vi "Accelerator Not Complex Process.vi"(9 "Sessions Parameters":T2={"intra_op_num_threads"=0, "inter_op_num_threads"=0, "execution_mode"=enum."ORT_SEQUENTIAL", "deterministic_compute"=FALSE, "graph_optimization_level"=1, "optimized_model_file_path"=path "", "profiling output dir"=path ""} {"graph_optimization_level" items=["ORT_DISABLE_ALL"=0, "ORT_ENABLE_ALL"=1, "ORT_ENABLE_BASIC"=2, "ORT_ENABLE_EXTENDED"=99]}, 10 "Execution Device":T1=enum."CUDA", 11 "X size":i32=16384) -> (3 "Accelerator Time":dbl=1.5238084999999728)   [LabVIEW 2020]
uses:
  Source/_Controls/acc_execution_provider_enum.ctl
  Source/ONNX/_Controls/acc_CUDA_ep_params_simplified.ctl
  Source/ONNX/_Controls/acc_tensorRT_ep_params_simplified.ctl
  Source/ONNX/Inference/acc_Inference.lvclass/acc_Inference.ctl
  Source/ONNX/Inference/_Methods/Simplified/acc_embedded_run_preallocated_multi_input_and_outputs_gpu_by_idx.vi
  Source/ONNX/Inference/_Methods/Simplified/acc_embedded_copy_ptr_data_to_labview_data.vi
  Source/ONNX/Inference/_Methods/Simplified/acc_embedded_run_mono_output_scalar_float.vi
  Source/SubVIs/sort_array/acc_sort_1d_index_ptr_data_cluster_array.vi
  Source/ONNX/Inference/_Methods/acc_embedded_run_preallocated_inputs_outputs_cuda_store_local.vi
  Source/SubVIs/sort_array/acc_sort_1d_index_out_ptr_data_cluster_array.vi
  Source/SubVIs/CUDAFunctions/acc_cuda_memcpy_device_to_host_bytes.vi
  Source/SubVIs/CUDAFunctions/acc_cuda_check_error.vi
  Source/SubVIs/CUDAFunctions/acc_cuda_error.vi
  Source/ONNX/Inference/acc_Inference.lvclass
  C:/Users/COCO/TDF Dropbox/1_Graiphic/3 - Services et Etudes/2 - Dev/code/Toolkits/Accelerator/Source/ONNX/acc_ONNX.lvclass
  Source/SubVIs/add_to_cluster_onnx_input/acc_onnx_add_1d_float_array_into_ptr_input_cluster_array_by_idx.vi
  Source/Model/_Methods/acc_create_onnx_model_then_init_cuda_inference_session.vi
  Source/Model/_Methods/acc_create_onnx_model_then_init_inference_session.vi
  Source/Model/_Methods/acc_create_onnx_model_then_init_tensorRT_inference_session.vi
  Source/SubVIs/add_to_cluster_onnx_input/acc_onnx_add_scalar_float_array_into_ptr_input_cluster_array_by_idx.vi
  Source/ONNX/Inference/_Methods/acc_embedded_check_execution_inputs_index.vi
  Source/ONNX/Inference/_Methods/acc_embedded_check_execution_outputs_index.vi
  Source/ONNX/_Accessors/acc_Read dll_path.vi
  Source/ONNX/SubVIs/acc_ONNX_CheckError.vi
  Source/SubVIs/CUDAFunctions/cuda_path_without_check_version.vi
  Source/SubVIs/Acc_ErrorStop.vi
  Source/SubVIs/checks/acc_check_output_onnx.vi
  Source/Model/acc_Model.lvclass
  <vilib>/Analysis/NI_AALBase.lvlib
panel:
  in  "nb_loop":i32=6
  out "max value":sgl=1.3257894e+20
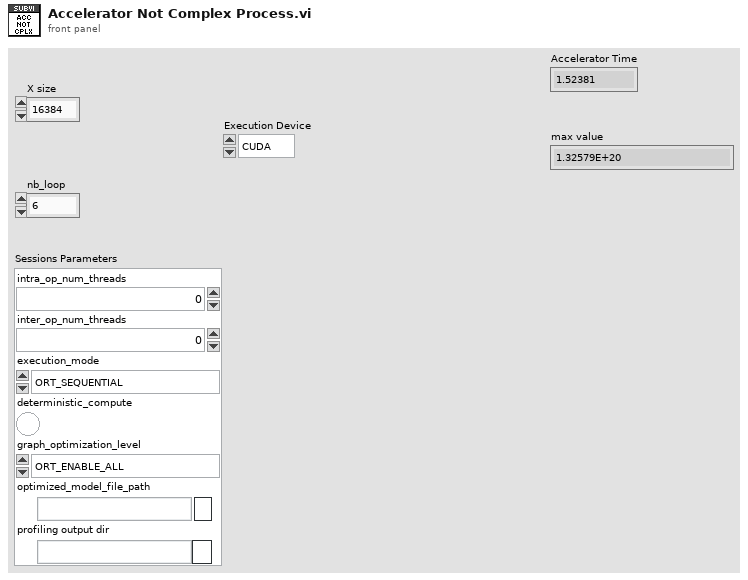
[diagram p1: front panel]
types:
  T1 = typedef "acc_execution_provider_enum.ctl" = enum16{"CPU", "CUDA", "TensorRT"}
  T2 = cluster{"intra_op_num_threads":i32, "inter_op_num_threads":i32, "execution_mode":enum16{"ORT_SEQUENTIAL", "ORT_PARALLEL"}, "deterministic_compute":bool, "graph_optimization_level":u16, "optimized_model_file_path":path, "profiling output dir":path}
  T3 = typedef "acc_onnx_multi_ptr_input_index_cluster.ctl" = cluster{"input_order":u32, "Inputs Info":cluster{"inputs_ptr":u64, "inputs_shapes":i64[], "inputs_ranks":i64, "inputs_types":T4}}
  T4 = typedef "acc_onnx_dtype_enum.ctl" = enum16{"UNDEFINED", "FLOAT", "UINT8", "INT8", "UINT16", "INT16", "INT32", "INT64", "STRING", "BOOL", "FLOAT16", "DOUBLE", "UINT32", "UINT64", "COMPLEX64", "COMPLEX128", "BFLOAT16", "FLOAT8E4M3FN", "FLOAT8E4M3FNUZ", "FLOAT8E5M2", "FLOAT8E5M2FNUZ", "UINT4", "INT4"}
  T5 = typedef "acc_CUDA_ep_params_simplified.ctl" = cluster{"Device & Stream":cluster{"Device Index":i32, "Use Custom Compute Stream?":bool, "Custom Compute Stream (Pointer)":u64, "Copy Using Default Stream?":bool}, "Memory Management":cluster{"GPU Memory Limit (Bytes)":u64, "Arena Extension Strategy":enum16{"kNextPowerOfTwo", "kSameAsRequested"}, "Default Memory Arena Config":u64}, "CuDNN & Kernel Optimization":cluster{"cuDNN Convolution Algorithm Search":enum16{"OrtCudnnConvAlgoSearchExhaustive", "OrtCudnnConvAlgoSearchHeuristic", "OrtCudnnConvAlgoSearchDefault"}, "Use Max Workspace for cuDNN?":bool, "Pad Conv1D Inputs to NC1D?":bool, "Fuse Convolution + Bias?":bool, "Scaled Dot-Product Attention Kernel Option":bool, "Enable Strict SkipLayerNorm Mode?":bool}, "Execution & Precision Controls":cluster{"Enable CUDA Graph Execution?":bool, "Use EP-Level Unified Stream?":bool, "Prefer NHWC Tensor Layout?":bool, "Use TensorFloat-32 (TF32)?":bool}, "Tunable Operator System":cluster{"Enable Tunable Operators?":bool, "Enable Tuning Mode for Tunable Operators?":bool, "Max Tuning Duration (ms)":i32}}
  T6 = typedef "acc_tensorRT_ep_params_simplified.ctl" = cluster{"Device And Stream":cluster{"Device Index":i32, "Use Custom Compute Stream?":bool, "Custom Compute Stream (Pointer)":u64}, "Parser & Subgraph Options":cluster{"Max Partition Attemps":i32, "Minimum Subgraph Size":i32}, "Memory & Workspace Management":cluster{"Max Workspace Memory (Bytes)":u64, "Share Memory Between Subgraphs":bool, "Auxiliary Stream Count":i32}, "Precision & Numeric Modes":cluster{"Enable FP16":bool, "Enable BF16":bool, "Enable INT8":bool, "INT8 Calibration Table Name":path, "Use Native INT8 Calibration?":bool}, "Engine Build, Cache & Paths":cluster{"Enable Engine Caching?":bool, "Engine Cache Directory":path, "Enable Engine Decryption?":bool, "Decryption Library Path":path, "Build Engines Sequentially?":bool, "Enable Timing Cache?":bool, "Timing Cache Directory":path, "Force Timing Cache Use?":bool, "Enable Detailed Logs?":bool, "Use Build Heuristics?":bool, "Enable Weight Sparsity?":bool, "Engine Optimization Level (0–5)":i32}, "Paths & Plugins":cluster{"Extra Plugin Libraries":path[], "Tactic Source Rules":string, "Enabled Preview Features":enum16{"None", "ALIASED_PLUGIN_IO_10_03"}}, "Profile Shapes":cluster{"Minimum Input Shapes":string, "Maximum Input Shapes":string, "Optimal Input Shapes":string}, "Advanced & DLA / CUDA Graph":cluster{"Enable DLA Acceleration?":bool, "DLA Core Index":i32, "Dump TensorRT Subgraphs?":bool, "Force LayerNorm in FP32?":bool, "Enable CUDA Graph Execution?":bool}}
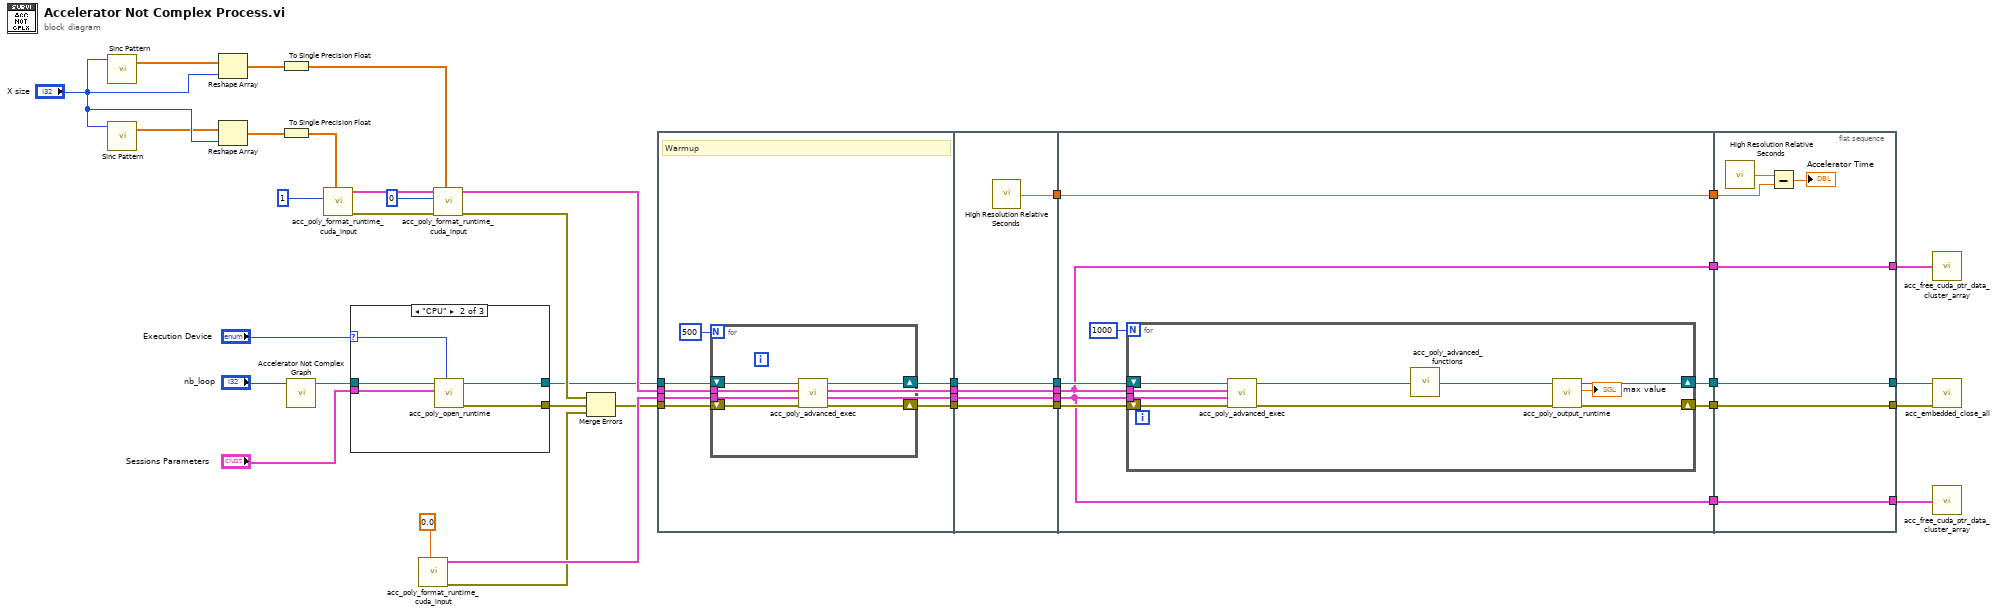
[diagram p0: block diagram]
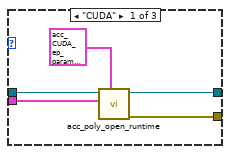
[diagram p2: hidden frame]
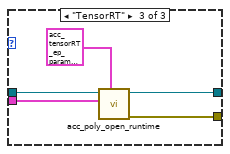
[diagram p3: hidden frame]
diagram:
  n1 = call <vilib>:"Sinc Pattern.vi"("samples"="X size") -> ("Sinc Pattern"=w8:dbl[])  [unwired: 3 in, 1 out]
  n2 = call <vilib>:"Sinc Pattern.vi"("samples"="X size") -> ("Sinc Pattern"=w9:dbl[])  [unwired: 3 in, 1 out]
  n3 = Reshape Array(w8, "X size") -> (w7:dbl[])
  n4 = Reshape Array(w9, "X size") -> (w6:dbl[])
  n5 = To Single Precision Float(number=w7) -> (single precision float=w10:sgl[])
  n6 = To Single Precision Float(number=w6) -> (single precision float=w11:sgl[])
  n7 = call "Accelerator Not Complex Graph.vi"("nb_loop"="nb_loop") -> ("Model out"=w3:refnum<class "acc_Model.lvclass">)  [unwired: 10 in]
  n8 = call-poly "acc_poly_format_runtime_cuda_input.vi"("1D Input Data"=w11, "input order"=1) -> ("error out"=w31:errorcluster, "Data in"=w36:T3[])  [unwired: 8 in]
  n9 = case shown="\"CPU\"" "Execution Device" {
    selector: "Execution Device" -> [_ w47 _]
    tunnel: [w46 w51 w56] -> w5
    tunnel: [w45 w50 w55] -> w1
    tunnel: "Sessions Parameters" -> [w44 w49 w54]
    tunnel: w3 -> [w43 w48 w53]
    frame "CUDA" {
      n10 = call-poly "acc_poly_open_runtime.vi"("CUDA Parameters"=T5 {"Device & Stream"={"Device Index"=0, "Use Custom Compute Stream?"=FALSE, "Custom Compute Stream (Pointer)"=0, "Copy Using Default Stream?"=TRUE}, "Memory Management"={"GPU Memory Limit (Bytes)"=18446744073709551615, "Arena Extension Strategy"=enum."kSameAsRequested", "Default Memory Arena Config"=0}, "CuDNN & Kernel Optimization"={"cuDNN Convolution Algorithm Search"=enum."OrtCudnnConvAlgoSearchHeuristic", "Use Max Workspace for cuDNN?"=FALSE, "Pad Conv1D Inputs to NC1D?"=FALSE, "Fuse Convolution + Bias?"=FALSE, "Scaled Dot-Product Attention Kernel Option"=FALSE, "Enable Strict SkipLayerNorm Mode?"=FALSE}, "Execution & Precision Controls"={"Enable CUDA Graph Execution?"=TRUE, "Use EP-Level Unified Stream?"=FALSE, "Prefer NHWC Tensor Layout?"=FALSE, "Use TensorFloat-32 (TF32)?"=TRUE}, "Tunable Operator System"={"Enable Tunable Operators?"=FALSE, "Enable Tuning Mode for Tunable Operators?"=FALSE, "Max Tuning Duration (ms)"=0}}, "Sessions Parameters"=w44, "Model in"=w43) -> ("error out"=w45:errorcluster, "Inference out"=w46:refnum<class "acc_Inference.lvclass">)  [unwired: 7 in]
    }
    frame "CPU" {
      n11 = call-poly "acc_poly_open_runtime.vi"("Execution Device"=w47, "Sessions Parameters"=w49, "Model in"=w48) -> ("error out"=w50:errorcluster, "Inference out"=w51:refnum<class "acc_Inference.lvclass">)  [unwired: 7 in]
    }
    frame "TensorRT" {
      n12 = call-poly "acc_poly_open_runtime.vi"("TRT Parameters"=T6 {"Device And Stream"={"Device Index"=0, "Use Custom Compute Stream?"=FALSE, "Custom Compute Stream (Pointer)"=0}, "Parser & Subgraph Options"={"Max Partition Attemps"=1000, "Minimum Subgraph Size"=1}, "Memory & Workspace Management"={"Max Workspace Memory (Bytes)"=0, "Share Memory Between Subgraphs"=FALSE, "Auxiliary Stream Count"=-1}, "Precision & Numeric Modes"={"Enable FP16"=FALSE, "Enable BF16"=FALSE, "Enable INT8"=FALSE, "INT8 Calibration Table Name"=path "", "Use Native INT8 Calibration?"=FALSE}, "Engine Build, Cache & Paths"={"Enable Engine Caching?"=FALSE, "Engine Cache Directory"=path "", "Enable Engine Decryption?"=FALSE, "Decryption Library Path"=path "", "Build Engines Sequentially?"=FALSE, "Enable Timing Cache?"=FALSE, "Timing Cache Directory"=path "", "Force Timing Cache Use?"=FALSE, "Enable Detailed Logs?"=FALSE, "Use Build Heuristics?"=FALSE, "Enable Weight Sparsity?"=FALSE, "Engine Optimization Level (0–5)"=3}, "Paths & Plugins"={"Extra Plugin Libraries"=[], "Tactic Source Rules"="", "Enabled Preview Features"=enum."None"}, "Profile Shapes"={"Minimum Input Shapes"="", "Maximum Input Shapes"="", "Optimal Input Shapes"=""}, "Advanced & DLA / CUDA Graph"={"Enable DLA Acceleration?"=FALSE, "DLA Core Index"=0, "Dump TensorRT Subgraphs?"=FALSE, "Force LayerNorm in FP32?"=FALSE, "Enable CUDA Graph Execution?"=FALSE}}, "Sessions Parameters"=w54, "Model in"=w53) -> ("error out"=w55:errorcluster, "Inference out"=w56:refnum<class "acc_Inference.lvclass">)  [unwired: 7 in]
    }
  }
  n13 = call-poly "acc_poly_format_runtime_cuda_input.vi"("Input Data"=sgl 0.0) -> ("error out"=w15:errorcluster, "Data in"=w34:T3[])  [unwired: 9 in]
  n14 = call-poly "acc_poly_format_runtime_cuda_input.vi"("1D Input Data"=w10, "error in"=w31, "input order"=0, "Data in"=w36) -> ("error out"=w16:errorcluster, "Data in"=w35:T3[])  [unwired: 6 in]
  n15 = Merge Errors(w16, w1, w15) -> (w29:errorcluster)
  n16 = flat-sequence {
    tunnel: w29 -> [w62]
    tunnel: w35 -> [w61]
    tunnel: w34 -> [w60]
    tunnel: [w63] -> w22
    tunnel: [w61] -> w21
    tunnel: [w60] -> w20
    tunnel: [w59] -> w19
    tunnel: w5 -> [w57]
    tunnel: [w74] -> w41
    tunnel: [w73] -> w39
    tunnel: [w72] -> w33
    tunnel: [w71] -> w32
    tunnel: [w70] -> w30
    tunnel: w22 -> [w73]
    tunnel: w21 -> [w71]
    tunnel: w20 -> [w72]
    tunnel: w19 -> [w70]
    tunnel: w41 -> [w82]
    tunnel: [w82] -> w40
    tunnel: w39 -> [w80]
    tunnel: w33 -> [w75]
    tunnel: w32 -> [w76]
    tunnel: w30 -> [w79]
    tunnel: [w78] -> w27
    tunnel: [w77] -> w26
    tunnel: [w76] -> w24
    tunnel: [w75] -> w23
    tunnel: w40 -> [w98]
    tunnel: [w96] -> w28
    tunnel: w27 -> [w96]
    tunnel: w26 -> [w95]
    tunnel: [w95] -> w25
    tunnel: [w94] -> w14
    tunnel: w24 -> [w94]
    tunnel: [w93] -> w13
    tunnel: w23 -> [w93]
    frame #0 {
      # "Warmup"
      n17 = for {
        N: 500 -> [_]
        tunnel: w61 -> [w66]
        tunnel: w60 -> [w65]
        shift-right: [w68] -> w63
        shift-left: w57 -> [w69]
        shift-right: [w64] -> w59
        shift-left: w62 -> [w67]
        n18 = call-poly "acc_poly_advanced_exec.vi"("error in"=w67, "Data out"=w65, "Data in"=w66, "Inference in"=w69) -> ("error out"=w64:errorcluster, "Inference out"=w68:refnum<class "acc_Inference.lvclass">)  [unwired: 6 in]
      }
    }
    frame #1 {
      n19 = call <vilib>:"High Resolution Relative Seconds.vi"() -> ("relative seconds"=w74:dbl)
    }
    frame #2 {
      n20 = for {
        N: 1000 -> [_]
        tunnel: w75 -> [w91]
        tunnel: w76 -> [w90]
        shift-right: [w86] -> w78
        shift-left: w80 -> [w92]
        shift-right: [w85] -> w77
        shift-left: w79 -> [w89]
        n21 = call-poly "acc_poly_advanced_exec.vi"("error in"=w89, "Data out"=w91, "Data in"=w90, "Inference in"=w92) -> ("error out"=w87:errorcluster, "Inference out"=w88:refnum<class "acc_Inference.lvclass">)  [unwired: 6 in]
        n22 = call-poly "acc_poly_advanced_functions.vi"("Inference in"=w88) -> ("Inference out"=w84:refnum<class "acc_Inference.lvclass">)
        n23 = call-poly "acc_poly_output_runtime.vi"("error in"=w87, "Inference in"=w84) -> ("error out"=w85:errorcluster, "Output Data"=→"max value":sgl, "Inference out"=w86:refnum<class "acc_Inference.lvclass">)  [unwired: 7 in]
      }
    }
    frame #3 {
      n24 = call <vilib>:"High Resolution Relative Seconds.vi"() -> ("relative seconds"=w99:dbl)
      n25 = Subtract(x=w99, y=w98) -> (x-y=→"Accelerator Time":dbl)
    }
  }
  n26 = call "acc_free_cuda_ptr_data_cluster_array.vi"("Data in"=w14) -> ()
  n27 = call-dynamic "acc_embedded_close_all.vi"("error in"=w25, "Inference in"=w28) -> ()  [unwired: 8 in, 2 out]
  n28 = call "acc_free_cuda_ptr_data_cluster_array.vi"("Data in"=w13) -> ()
